vi "AGCxxx Close.vi"(0 "AGCxxx VISA Cluster":T1={"VISA resource name"="", "VISA Timeout Value (1000 ms)"=1000, "Lock Timeout (1000 ms)"=1000, "MAX Channel (6)"=6}, 11 "error in (no error)":errorcluster) -> (15 "error out":errorcluster)   [LabVIEW 2014, in "AGCxxx - Driver.lvlib"]
doc: "This VI closes the I/O interface with the instrument.\n\nCopyright (C) \nGesellschaft f. Schwerionenforschung, GSI\nPlanckstr. 1\n64291 Darmstadt\nGermany\n\nContact: http://www-wnt.gsi.de/labview\n H.Brand@gsi.de\n\nThis program is free software; you can redistribute it and/or\nmodify it under the terms of the GNU General Public License\nas published by the Free Software Foundation; either version 2\nof the License, or (at your option) any later version.\n\nThis program is distributed in the hope that it will be useful,\nbut WITHOUT ANY WARRANTY; without even the implied warranty of\nMERCHANTABILITY or FITNESS FOR A PARTICULAR PURPOSE. See the\nGNU General Public License for more details (http://www.gnu.org)."
uses:
  AGCxxx - Driver.lvlib
  AGCxxx VISA Control.ctl
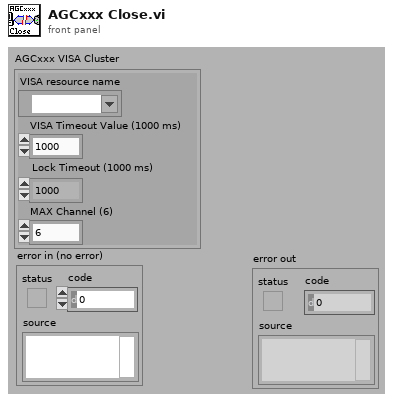
[diagram p1: front panel]
types:
  T1 = typedef "AGCxxx - Driver.lvlib/AGCxxx VISA Control.ctl" = cluster{"VISA resource name":refnum<visa-resource-name>, "VISA Timeout Value (1000 ms)":u32, "Lock Timeout (1000 ms)":u32, "MAX Channel (6)":i32}
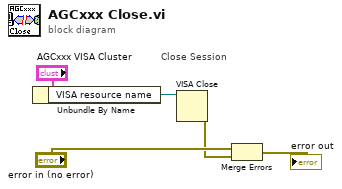
[diagram p0: block diagram]
diagram:
  # "Close Session"
  n1 = Unbundle By Name("AGCxxx VISA Cluster") -> ("VISA resource name"=w4:refnum<visa-resource-name>)
  n2 = VISA Close(VISA resource name=w4) -> (error out=w2:errorcluster)  [unwired: 1 in]
  n3 = Merge Errors("error in (no error)", w2) -> (→"error out":errorcluster)
